vi "RetaInimigoBolaUsandoOrientacao.vi"(0 "Y quina":dbl format="%#_13g", 4 "Goal Width":u32, 5 "Field length":u32, 7 "Meio?":bool=TRUE, 8 "Orientação inimigo":dbl format="%#_13g", 10 "Y bola":dbl format="%#_13g", 11 "X bola":dbl format="%#_13g") -> (1 "Orientação goleiro":dbl format="%#_13g", 2 "Y golerio":dbl format="%#_13g", 3 "X goleiro":dbl format="%#_13g")   [LabVIEW 2020]
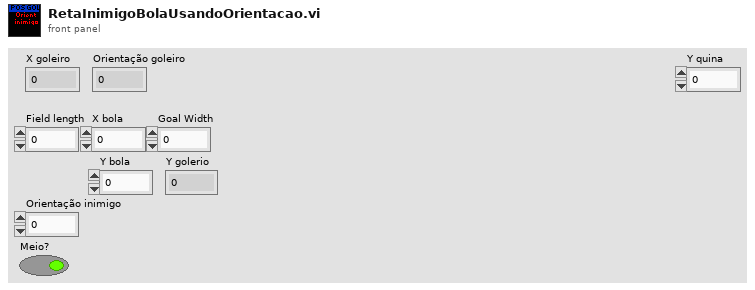
[diagram p1: front panel]
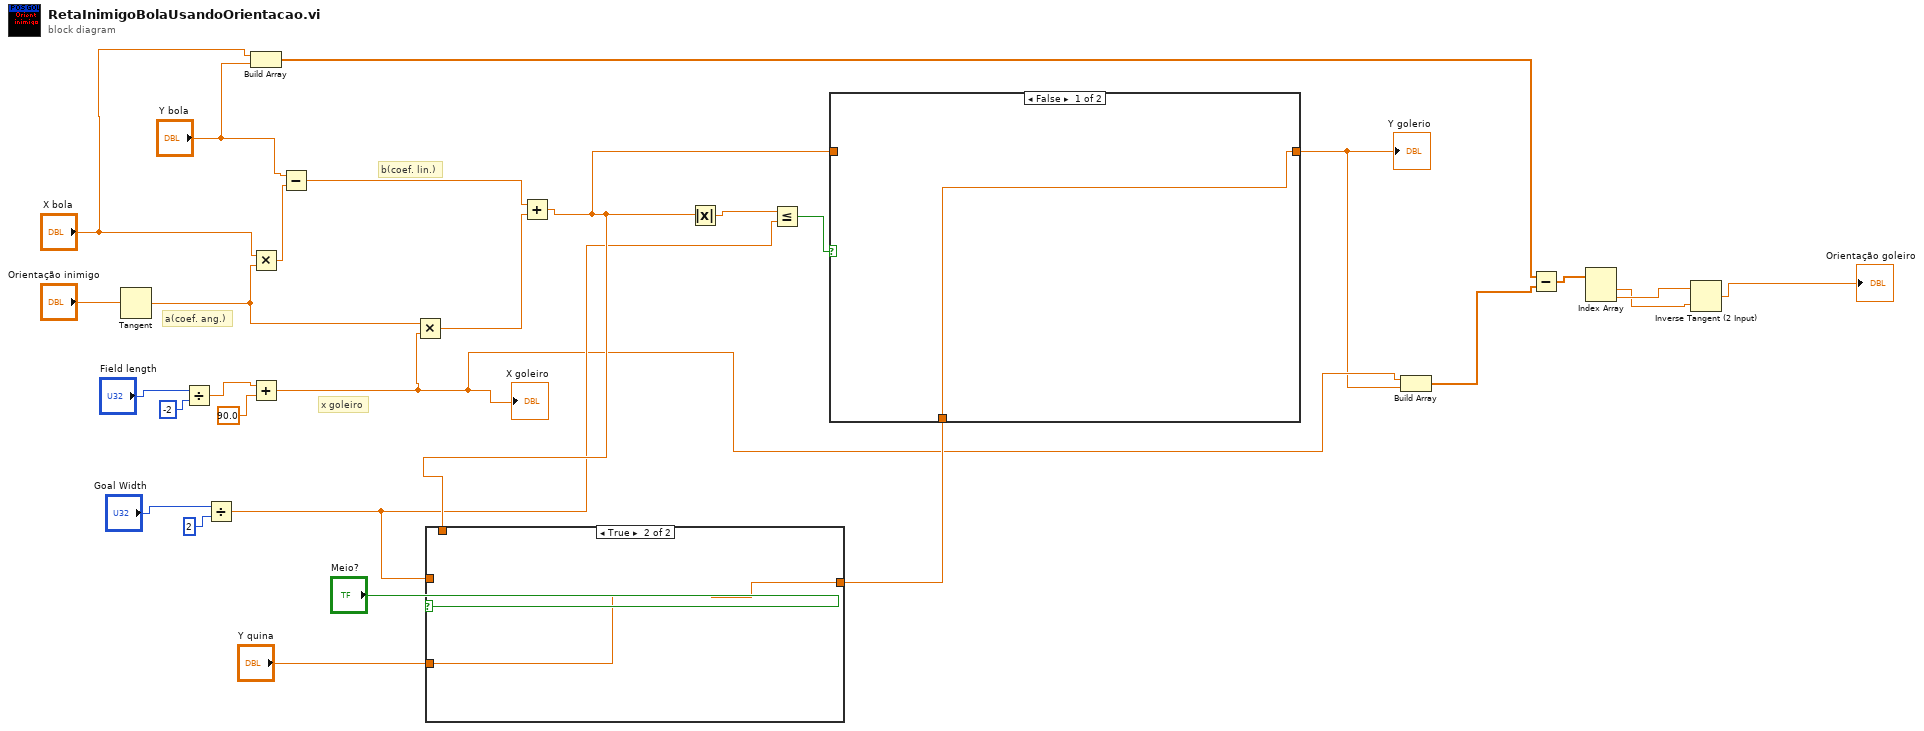
[diagram p0: block diagram]
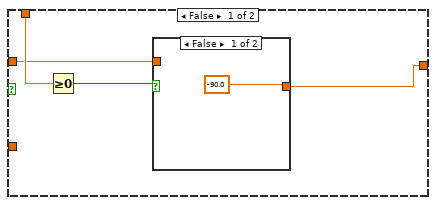
[diagram p2: hidden frame]
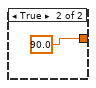
[diagram p3: hidden frame]
diagram:
  # "b(coef. lin.)"
  # "x goleiro"
  # "a(coef. ang.)"
  n1 = Tangent(1:"Orientação inimigo") -> (0:w23:dbl)
  n2 = Divide(x="Field length", y=-2) -> (x/y=w25:dbl)
  n3 = Divide(x="Goal Width", y=2) -> (x/y=w13:dbl)
  n4 = Build Array("X bola", "Y bola") -> (w6:dbl[])
  n5 = Multiply(x="X bola", y=w23) -> (x*y=w28:dbl)
  n6 = Add(x=w25, y=90.0 ("x+y")) -> (x+y=w10:dbl)
  "X goleiro" <- w10
  n7 = Subtract(x="Y bola", y=w28) -> (x-y=w22:dbl)
  n8 = Multiply(x=w23, y=w10) -> (x*y=w21:dbl)
  n9 = Add(x=w22, y=w21) -> (x+y=w14:dbl)
  n10 = case shown="True" "Meio?" {
    tunnel: [w29 w35] -> w15
    tunnel: w14 -> [w32 _]
    tunnel: w13 -> [w30 _]
    tunnel: "Y quina" -> [_ w35]
    frame False {
      n11 = Greater Or Equal To 0?(x=w32) -> (x >= 0?=w31:bool)
      n12 = case shown="False" w31 {
        tunnel: w30 -> [_ _]
        tunnel: [-90.0 ("y") 90.0 ("y")] -> w29
        frame False {
        }
        frame True {
        }
      }
    }
    frame True {
    }
  }
  n13 = Absolute Value(x=w14) -> (abs(x)=w18:dbl)
  n14 = Less Or Equal?(x=w18, y=w13) -> (x <= y?=w17:bool)
  n15 = case shown="False" w17 {
    tunnel: [w36 w37] -> w9
    tunnel: w14 -> [_ w37]
    tunnel: w15 -> [w36 _]
    frame False {
    }
    frame True {
    }
  }
  "Y golerio" <- w9
  n16 = Build Array(w10, w9) -> (w5:dbl[])
  n17 = Subtract(x=w6, y=w5) -> (x-y=w4:dbl[])
  n18 = Index Array(array=w4) -> (element #1=w2:dbl, element #2=w3:dbl)  [unwired: 2 in]
  n19 = Inverse Tangent (2 Input)(1:w2, 2:w3) -> (0:→"Orientação goleiro":dbl)
